vi "AudioTest.Create Mic Level and Attenuation Result.vi"(4 "Delta LL":dbl format="%.2f", 6 "Delta":dbl format="%.2f", 8 "Level UL":dbl format="%.2f", 9 "Level LL":dbl format="%.2f", 10 "Level":dbl format="%.2f", 11 "Side":string="Left") -> (0 "Delta Color":u32(colorbox), 1 "Level Color":u32(colorbox), 3 "Data":T1[](array[typedef]) {"Status" items=["LOG", "PASS", "FAIL", "ERROR"]})   [LabVIEW 2018]
uses:
  Common/Utils/Results/Result.Measurement Item.ctl
  Common/Utils/Results/Result.Measurement and Attribute Item Status.ctl
  Common/Utils/Results/Result.Limit Type.ctl
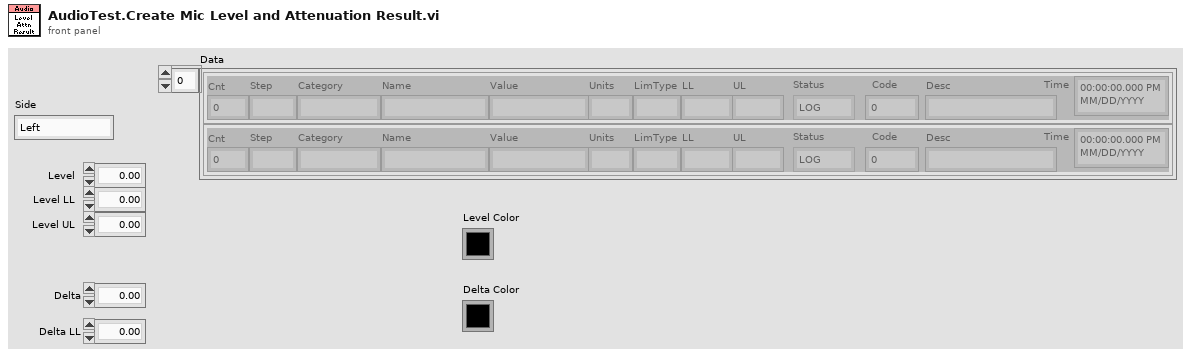
[diagram p1: front panel]
types:
  T1 = typedef "Result.Measurement Item.ctl" = cluster{"Cnt":i32, "Step":string, "Category":string, "Name":string, "Value":string, "Units":string, "LimType":string, "LL":string, "UL":string, "Status":T2, "Code":i32, "Desc":string, "Time":timestamp}
  T2 = typedef "Result.Measurement and Attribute Item Status.ctl" = i32
  T3 = typedef "Result.Limit Type.ctl" = enum16{"None", "EQ", "NE", "GT", "LT", "GE", "LE", "GTLT", "GELE", "GELT", "GTLE", "LTGT", "LEGE", "LEGT", "LTGE", "Contains", "NotContains"}
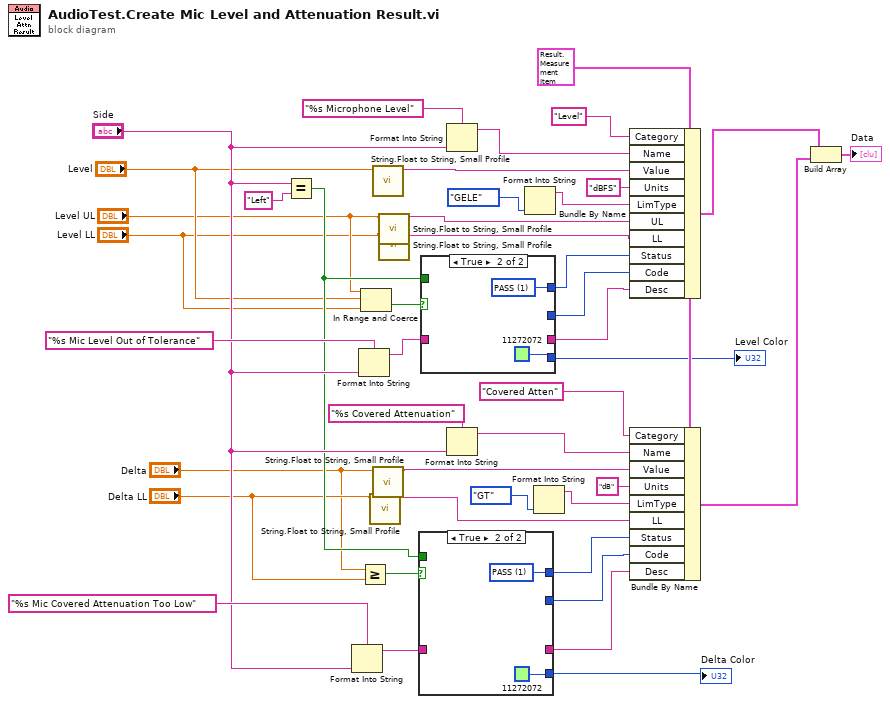
[diagram p0: block diagram]
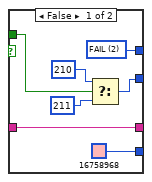
[diagram p2: hidden frame]
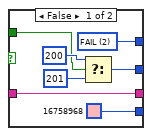
[diagram p3: hidden frame]
diagram:
  w38 = T1 {"Cnt"=0, "Step"="", "Category"="", "Name"="", "Value"="", "Units"="", "LimType"="", "LL"="", "UL"="", "Status"=0, "Code"=0, "Desc"="", "Time"=timestamp(0 s since 1904-01-01)} ("Meas")
  n1 = Equal?(x="Side", y="Left") -> (x = y?=w18:bool)
  n2 = Format Into String(format string="%s Mic Covered Attenuation Too Low" ("Category"), "Side") -> (resulting string=w22:string)  [unwired: 2 in, 1 out]
  n3 = Format Into String(format string="%s Mic Level Out of Tolerance" ("Category"), "Side") -> (resulting string=w27:string)  [unwired: 2 in, 1 out]
  n4 = Greater Or Equal?(x="Delta", y="Delta LL") -> (x >= y?=w21:bool)
  n5 = In Range and Coerce(upper limit="Level UL", x="Level", lower limit="Level LL") -> (In Range?=w34:bool)  [unwired: 1 out]
  n6 = call "String.Float to String, Small Profile.vi"("Numeric"="Delta LL") -> ("String"=w6:string)  [unwired: 10 in]
  n7 = call "String.Float to String, Small Profile.vi"("Numeric"="Level") -> ("String"=w14:string)  [unwired: 10 in]
  n8 = call "String.Float to String, Small Profile.vi"("Numeric"="Delta") -> ("String"=w5:string)  [unwired: 10 in]
  n9 = call "String.Float to String, Small Profile.vi"("Numeric"="Level UL") -> ("String"=w11:string)  [unwired: 10 in]
  n10 = call "String.Float to String, Small Profile.vi"("Numeric"="Level LL") -> ("String"=w12:string)  [unwired: 10 in]
  n11 = case shown="True" w21 {
    tunnel: [w50 w52] -> w25
    tunnel: [w46 _] -> w24
    tunnel: w22 -> [w49 _]
    tunnel: [w49 _] -> w23
    tunnel: w18 -> [w45 _]
    tunnel: [u32 16758968 u32 11272072] -> w16
    frame False {
      w50 = T2 2 items=["LOG", "PASS", "FAIL", "ERROR"] ("Status")
      n12 = Select(t=210, s=w45, f=211) -> (s? t:f=w46:i32)
    }
    frame True {
      w52 = T2 1 items=["LOG", "PASS", "FAIL", "ERROR"] ("Status")
    }
  }
  "Delta Color" <- w16
  n13 = case shown="True" w34 {
    tunnel: [w59 w61] -> w33
    tunnel: [w55 _] -> w28
    tunnel: w27 -> [w58 _]
    tunnel: [w58 _] -> w26
    tunnel: w18 -> [w54 _]
    tunnel: [u32 16758968 u32 11272072] -> w17
    frame False {
      w59 = T2 2 items=["LOG", "PASS", "FAIL", "ERROR"] ("Status")
      n14 = Select(t=200, s=w54, f=201) -> (s? t:f=w55:i32)
    }
    frame True {
      w61 = T2 1 items=["LOG", "PASS", "FAIL", "ERROR"] ("Status")
    }
  }
  "Level Color" <- w17
  n15 = Format Into String(format string="%s Microphone Level" ("Category"), "Side") -> (resulting string=w31:string)  [unwired: 2 in, 1 out]
  n16 = Format Into String(format string="%s Covered Attenuation" ("Category"), "Side") -> (resulting string=w35:string)  [unwired: 2 in, 1 out]
  n17 = Format Into String(Result.Limit_Type."GELE" ("LimType")) -> (resulting string=w3:string)  [unwired: 3 in, 1 out]
  n18 = Format Into String(Result.Limit_Type."GT" ("LimType")) -> (resulting string=w1:string)  [unwired: 3 in, 1 out]
  n19 = Bundle By Name(cluster=w38, "Category"="Level", "Name"=w31, "Value"=w14, "Units"="dBFS", "LimType"=w3, "UL"=w11, "LL"=w12, "Status"=w33, "Code"=w28, "Desc"=w26) -> (w39:T1)
  n20 = Bundle By Name(cluster=w38, "Category"="Covered Atten", "Name"=w35, "Value"=w5, "Units"="dB", "LimType"=w1, "LL"=w6, "Status"=w25, "Code"=w24, "Desc"=w23) -> (w41:T1)
  n21 = Build Array(w39, w41) -> (→"Data":T1[])
